vi "main.vi"() -> ()   [LabVIEW 2018]
uses:
  <vilib>/DAQmx/create/channels.llb/DAQmx Create Channel (DO-Digital Output).vi
  <vilib>/DAQmx/write.llb/DAQmx Write (Digital 1D Bool NChan 1Samp 1Line).vi
  <resource>/objmgr/daqmx.rc
panel:
  out "Connexion Status":string="Not connected"
  in  "stop":bool
  out "Bits":bool[](array[boolean])
  in  "Bit":i32
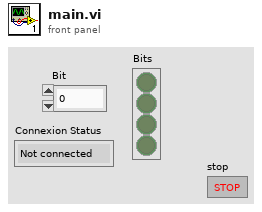
[diagram p1: front panel]
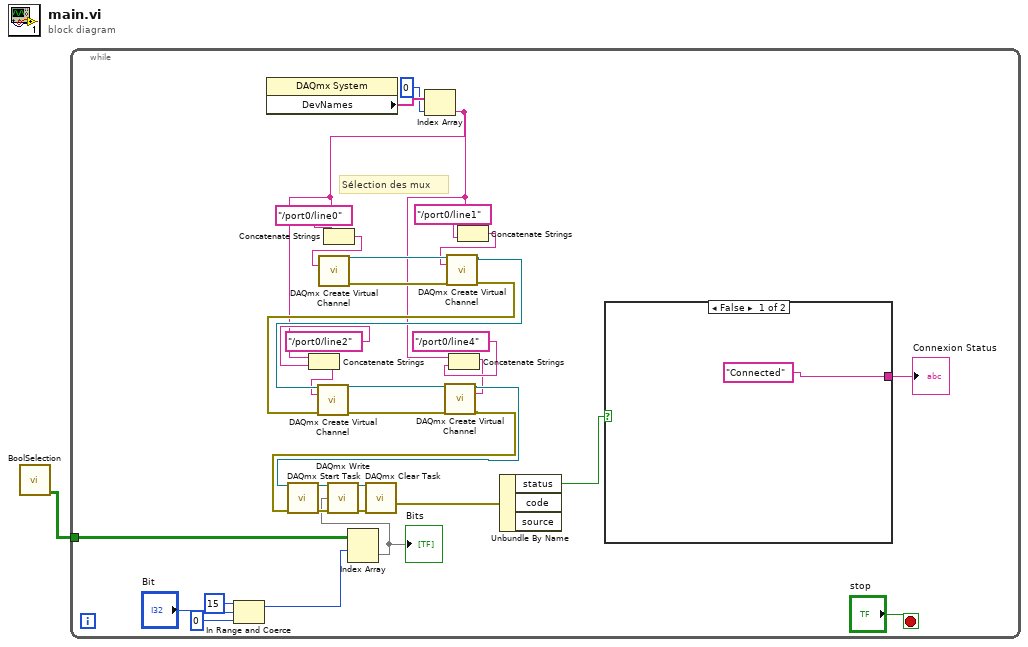
[diagram p0: block diagram]
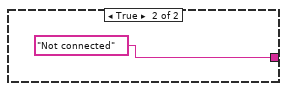
[diagram p2: hidden frame]
diagram:
  n1 = call "BoolSelection.vi"() -> ("BoolSelection"=w1:bool[][])  [unwired: 11 in]
  n2 = while {
    tunnel: w1 -> [w7]
    stop <- "stop" stop-if-true
    # "Sélection des mux"
    n3 = In Range and Coerce(upper limit=15, x="Bit", lower limit=0) -> (coerced(x)=w2:i32)  [unwired: 1 out]
    n4 = property class="DAQmx System"() -> ("DevNames"=w22:tag[])  [unwired: 2 in, 2 out]
    n5 = Index Array(array=w7, index (row)=w2) -> (element=w32:bool[])  [unwired: 1 in]
    "Bits" <- w32
    n6 = Index Array(array=w22, index=0) -> (element=w12:tag)
    n7 = Concatenate Strings(w12, "/port0/line2" ("string")) -> (w15:string)
    n8 = Concatenate Strings(w12, "/port0/line0" ("string")) -> (w20:string)
    n9 = call-poly <vilib>:"DAQmx Create Virtual Channel.vi"("lines"=w20) -> ("task out"=w28:refnum<k21>, "error out"=w29:errorcluster)  [unwired: 13 in]
    n10 = Concatenate Strings(w12, "/port0/line4" ("string")) -> (w13:string)
    n11 = Concatenate Strings(w12, "/port0/line1" ("string")) -> (w17:string)
    n12 = call-poly <vilib>:"DAQmx Create Virtual Channel.vi"("task in"=w28, "lines"=w17, "error in"=w29) -> ("task out"=w27:refnum<k21>, "error out"=w26:errorcluster)  [unwired: 11 in]
    n13 = call-poly <vilib>:"DAQmx Create Virtual Channel.vi"("task in"=w27, "lines"=w15, "error in"=w26) -> ("task out"=w24:refnum<k21>, "error out"=w25:errorcluster)  [unwired: 11 in]
    n14 = call-poly <vilib>:"DAQmx Create Virtual Channel.vi"("task in"=w24, "lines"=w13, "error in"=w25) -> ("task out"=w23:refnum<k21>, "error out"=w8:errorcluster)  [unwired: 11 in]
    n15 = call <vilib>:"DAQmx Start Task.vi"("task/channels in"=w23, "error in"=w8) -> ("task out"=w33:refnum<k21>, "error out"=w34:errorcluster)  [unwired: 12 in]
    n16 = call-poly <vilib>:"DAQmx Write.vi"("task/channels in"=w33, "data"=w32, "error in"=w34) -> ("task out"=w31:refnum<k21>, "error out"=w30:errorcluster)  [unwired: 10 in, 1 out]
    n17 = call <vilib>:"DAQmx Clear Task.vi"("task in"=w31, "error in"=w30) -> ("error out"=w5:errorcluster)  [unwired: 13 in]
    n18 = Unbundle By Name(w5) -> ("status"=w4:bool)  [unwired: 2 out]
    n19 = case shown="False" w4 {
      tunnel: ["Connected" "Not connected"] -> w3
      frame False {
      }
      frame True {
      }
    }
    "Connexion Status" <- w3
  }
